vi "get_guide_points.vi"(8 "error in (no error)":errorcluster, 11 "TrajectoryDL110413StraightLine in":refnum<class "TrajectoryDL110413StraightLine.lvclass">) -> (0 "error out":errorcluster, 2 "guide points":refnum<class "SpaceVector.lvclass">[](array[class]), 3 "TrajectoryDL110413StraightLine out":refnum<class "TrajectoryDL110413StraightLine.lvclass">)   [LabVIEW 2010, in "TrajectoryDL110413StraightLine.lvclass"]
uses:
  TrajectoryDL110413StraightLine.lvclass
  common/classes/SpaceVector/SpaceVector/SpaceVector.lvclass
  TrajectoryDL110413StraightLine.lvclass/TrajectoryDL110413StraightLine.ctl
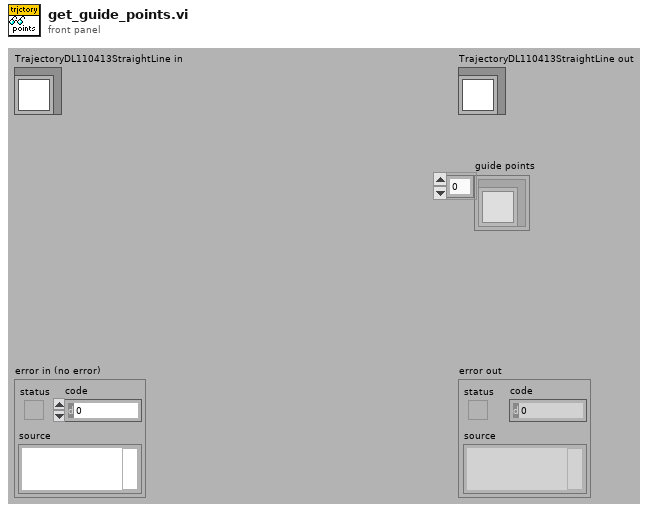
[diagram p1: front panel]
types:
  T1 = cluster{"Global Rectangle":dbl[unit][], "Contours":cluster{"Contour Type":u32, "ROI Type":u32, "Points":dbl[unit][]}[]}[]
  T2 = cluster{"Contour Type":u32, "ROI Type":u32, "Points":dbl[unit][]}[]
  T3 = cluster{"Points[0]":dbl[unit], "Points[1]":dbl[unit]}
  T4 = cluster{"Points[0]":dbl[unit], "Points[1]":dbl[unit], "Points[2]":dbl[unit], "Points[3]":dbl[unit]}
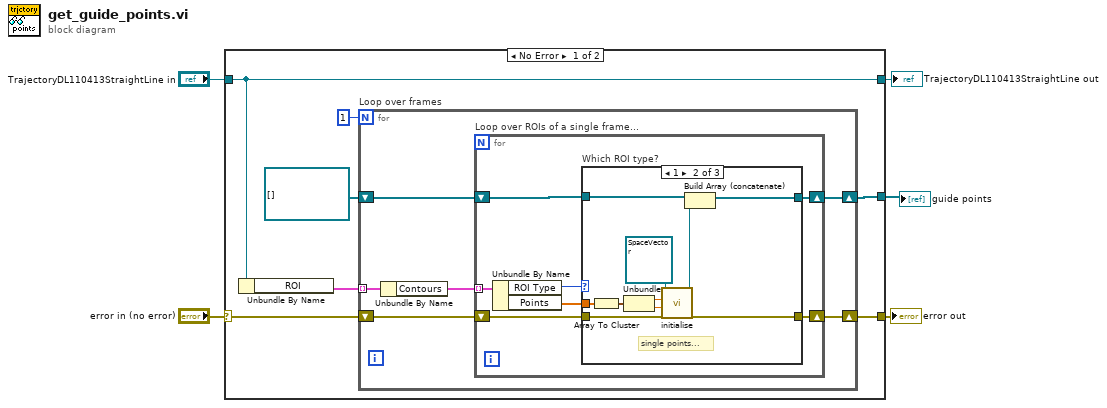
[diagram p0: block diagram]
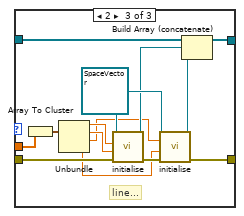
[diagram p3: hidden frame]
diagram:
  n1 = case shown="No Error" "error in (no error)" {
    selector: "error in (no error)" -> [w9 w53]
    tunnel: [w8 w53] -> w4
    tunnel: [w12 w52] -> w2
    tunnel: "TrajectoryDL110413StraightLine in" -> [w12 w52]
    tunnel: [w10 _] -> w1
    frame No Error {
      n2 = Unbundle By Name(w12) -> ("ROI"=w11:T1)
      n3 = for "Loop over frames" {
        N: 1 -> [_]
        tunnel: w11 -> [w18] mode=indexing
        shift-right: [w16] -> w8
        shift-left: w9 -> [w17]
        shift-right: [w13] -> w10
        shift-left: refnum<class "SpaceVector.lvclass">[] [] -> [w14]
        n4 = Unbundle By Name(w18) -> ("Contours"=w15:T2)
        n5 = for "Loop over ROIs of a single frame..." {
          shift-right: [w20] -> w16
          shift-left: w17 -> [w24]
          tunnel: w15 -> [w25] mode=indexing
          shift-right: [w23] -> w13
          shift-left: w14 -> [w22]
          n6 = Unbundle By Name(w25) -> ("ROI Type"=w19:u32, "Points"=w21:dbl[unit][])
          n7 = case "Which ROI type?" shown="1" w19 {
            tunnel: w21 -> [_ w37 w51]
            tunnel: w24 -> [w27 w35 w47]
            tunnel: [w27 w34 w45] -> w20
            tunnel: [w26 w31 w42] -> w23
            tunnel: w22 -> [w26 w30 w43]
            frame Default {
              # "not supported..."
            }
            frame 1 {
              # "single points..."
              n8 = Array To Cluster(array=w37) -> (cluster=w36:T3)
              n9 = Unbundle(w36) -> ("Points[0]"=w33:dbl[unit], "Points[1]"=w32:dbl[unit])
              n10 = call "initialise.vi"("error in (no error)"=w35, "y"=w32, "x"=w33, "SpaceVector in"=refnum<class "SpaceVector.lvclass"> refnum ("SpaceVector.lvclass")) -> ("error out"=w34:errorcluster, "SpaceVector out"=w28:refnum<class "SpaceVector.lvclass">)  [unwired: 6 in]
              n11 = Build Array (concatenate)(w30, w28) -> (w31:refnum<class "SpaceVector.lvclass">[])
            }
            frame 2 {
              w44 = refnum<class "SpaceVector.lvclass"> refnum ("SpaceVector.lvclass")
              # "line..."
              n12 = Array To Cluster(array=w51) -> (cluster=w50:T4)
              n13 = Unbundle(w50) -> ("Points[0]"=w49:dbl[unit], "Points[1]"=w48:dbl[unit], "Points[2]"=w38:dbl[unit], "Points[3]"=w39:dbl[unit])
              n14 = call "initialise.vi"("error in (no error)"=w47, "y"=w48, "x"=w49, "SpaceVector in"=w44) -> ("error out"=w46:errorcluster, "SpaceVector out"=w41:refnum<class "SpaceVector.lvclass">)  [unwired: 6 in]
              n15 = call "initialise.vi"("error in (no error)"=w46, "y"=w39, "x"=w38, "SpaceVector in"=w44) -> ("error out"=w45:errorcluster, "SpaceVector out"=w40:refnum<class "SpaceVector.lvclass">)  [unwired: 6 in]
              n16 = Build Array (concatenate)(w43, w41, w40) -> (w42:refnum<class "SpaceVector.lvclass">[])
            }
          }
        }
      }
    }
    frame Error {
    }
  }
  "error out" <- w4
  "TrajectoryDL110413StraightLine out" <- w2
  "guide points" <- w1
